vi "Microscope.CaptureImageAtCoords.vi"(6 "Move?":bool, 8 "error in (no error)":errorcluster, 9 "timeout (5000 ms)":i32=5000, 10 "Coords":T1, 11 "Microscope":refnum<class "Microscope.lvclass">) -> (0 "error out":errorcluster, 1 "Capture complete":bool, 2 "buffer":i32, 3 "Microscope out":refnum<class "Microscope.lvclass">)   [LabVIEW 2015, in "Microscope.lvclass"]
doc: "---------------------------------------------------------------\nJKI State Machine Objects™\nhttp://jki.net/state-machine-objects/\nCopyright (C) 2005-2015, JKI <info@jki.net>\nALL RIGHTS RESERVEDJKI State Machine Objects (SMO) 1.0.0.5\nJKI - JKI\nCopyright (c) 2016, JKI"
uses:
  Microscope.lvclass
  XYStage/Typedefs/(real)Coords--Cluster.ctl
  XYStage/XYStage.lvclass
  Camera/Camera.lvclass
panel:
  # "For instructions on how to use the JKI State Machine Objects, examples and video tutorials, visit:\nhttp://jki.net/state-machine-objects/\n\nJKI State Machine Objects™\nhttp://jki.net/state-machine-objects/\nCopyright (C) 2005-2015, JKI <info@jki.net>\nALL RIGHTS RESERVED"
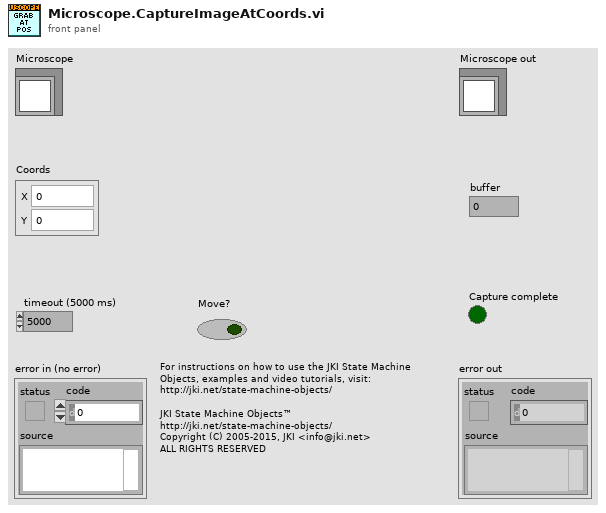
[diagram p1: front panel]
types:
  T1 = typedef "XYStage.lvclass/(real)Coords--Cluster.ctl" = cluster{"X":dbl, "Y":dbl}
  T2 = typedef "Microscope.lvclass/Dependencies--Cluster.ctl" = cluster{"XYStage":refnum<class "XYStage.lvclass">, "Camera":refnum<class "Camera.lvclass">}
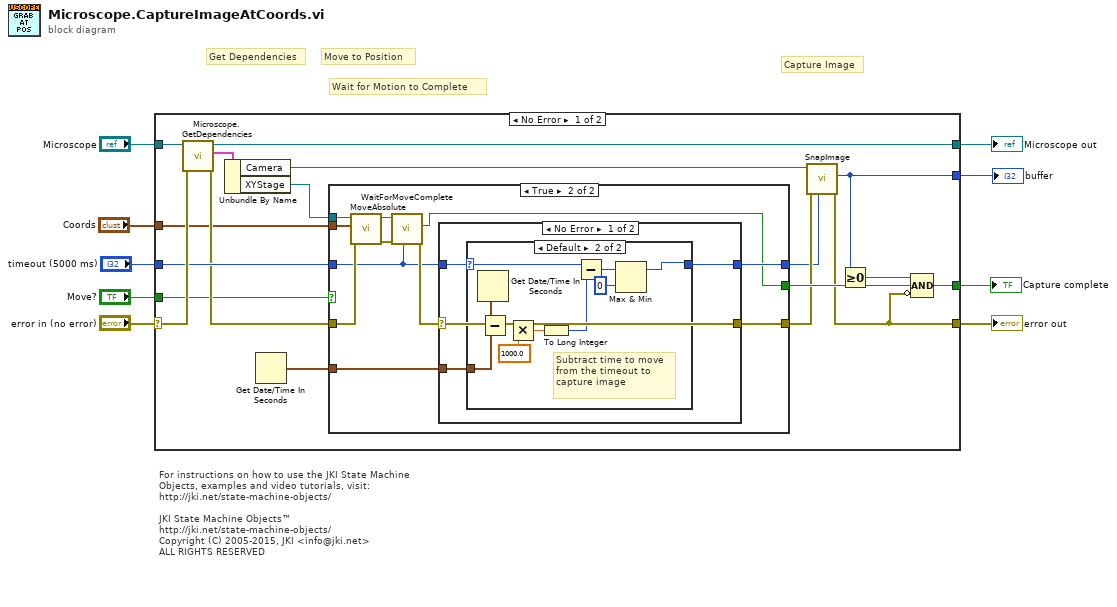
[diagram p0: block diagram]
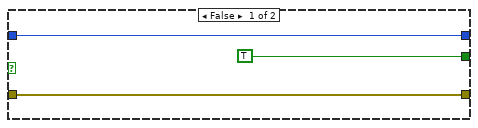
[diagram p2: hidden frame]
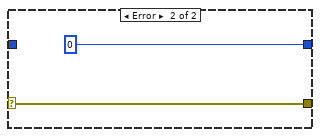
[diagram p4: hidden frame]
diagram:
  # "Capture Image"
  # "Wait for Motion to Complete"
  # "Move to Position"
  # "Get Dependencies"
  # "For instructions on how to use the JKI State Machine Objects, examples and video tutorials, visit:\nhttp://jki.net/state-machine-objects/\n\nJKI State Machine Objects™\nhttp://jki.net/state-machine-objects/\nCopyright (C) 2005-2015, JKI <info@jki.net>\nALL RIGHTS RESERVED"
  n1 = case shown="No Error" "error in (no error)" {
    selector: "error in (no error)" -> [w26 w59]
    tunnel: "Microscope" -> [w27 w60]
    tunnel: [w14 w59] -> w8
    tunnel: [w25 w60] -> w7
    tunnel: [w18 _] -> w4
    tunnel: "timeout (5000 ms)" -> [w23 _]
    tunnel: "Coords" -> [w20 _]
    tunnel: [w13 _] -> w2
    tunnel: "Move?" -> [w12 _]
    frame No Error {
      n2 = call "Microscope.GetDependencies.vi"("error in (no error)"=w26, "Microscope"=w27) -> ("error out"=w21:errorcluster, "Dependencies"=w24:T2, "Microscope out"=w25:refnum<class "Microscope.lvclass">)  [unwired: 7 in]
      n3 = Unbundle By Name(w24) -> ("Camera"=w17:refnum<class "Camera.lvclass">, "XYStage"=w22:refnum<class "XYStage.lvclass">)
      n4 = Get Date/Time In Seconds() -> (seconds since 1Jan1904=w11:timestamp)
      n5 = case shown="True" w12 {
        tunnel: w23 -> [w29 w34]
        tunnel: w22 -> [_ w41]
        tunnel: w21 -> [w28 w39]
        tunnel: w20 -> [_ w37]
        tunnel: [TRUE ("move complete") w31] -> w19
        tunnel: [w28 w33] -> w16
        tunnel: w11 -> [_ w32]
        tunnel: [w29 w35] -> w10
        frame False {
        }
        frame True {
          n6 = call "MoveAbsolute.vi"("error in (no error)"=w39, "Units"=w37, "XYStage"=w41) -> ("error out"=w38:errorcluster, "XYStage out"=w40:refnum<class "XYStage.lvclass">)  [unwired: 7 in]
          n7 = call "WaitForMoveComplete.vi"("timeout (5000 ms)"=w34, "error in (no error)"=w38, "XYStage"=w40) -> ("error out"=w36:errorcluster, "move complete"=w31:bool)  [unwired: 6 in, 1 out]
          n8 = case shown="No Error" w36 {
            selector: w36 -> [w45 w57]
            tunnel: [w42 0 ("timeout (5000 ms)")] -> w35
            tunnel: w34 -> [w43 _]
            tunnel: [w45 w57] -> w33
            tunnel: w32 -> [w44 _]
            frame No Error {
              n9 = case shown="Default" w43 {
                selector: w43 -> [w46 w51]
                tunnel: w44 -> [_ w56]
                tunnel: [w46 w48] -> w42
                frame ..-1 {
                }
                frame Default {
                  # "Subtract time to move\nfrom the timeout to\ncapture image"
                  n10 = Get Date/Time In Seconds() -> (seconds since 1Jan1904=w55:timestamp)
                  n11 = Subtract(x=w55, y=w56) -> (x-y=w54:dbl)
                  n12 = Multiply(x=w54, y=1000.0) -> (x*y=w52:dbl)
                  n13 = To Long Integer(number=w52) -> (32bit integer=w47:i32)
                  n14 = Subtract(x=w51, y=w47) -> (x-y=w50:i32)
                  n15 = Max & Min(x=w50, y=0) -> (max(x,y)=w48:i32)  [unwired: 1 out]
                }
              }
            }
            frame Error {
            }
          }
        }
      }
      n16 = call "SnapImage.vi"("timeout in ms (1000)"=w10, "error in (no error)"=w16, "Camera"=w17) -> ("error out"=w14:errorcluster, "buffer"=w13:i32)  [unwired: 6 in, 1 out]
      n17 = Greater Or Equal To 0?(x=w13) -> (x >= 0?=w15:bool)
      n18 = Compound Arithmetic op=AND(w15, w19, invert w14) -> (w18:bool)
    }
    frame Error {
    }
  }
  "error out" <- w8
  "Microscope out" <- w7
  "Capture complete" <- w4
  "buffer" <- w2
